vi "Create Spy.vi"(8 "error in (no error)":errorcluster) -> (0 "error out":errorcluster, 3 "LabSpy Out":refnum<data-value>)   [LabVIEW 2013, in "LabSpy.lvclass"]
doc: "Create a new spy object for use."
uses:
  LabSpy.lvclass
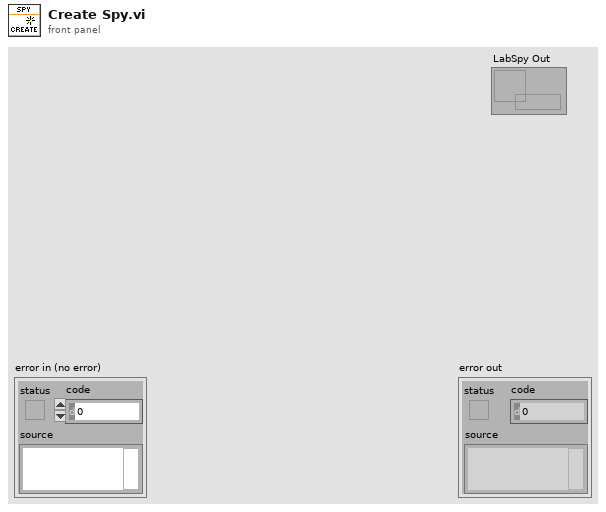
[diagram p1: front panel]
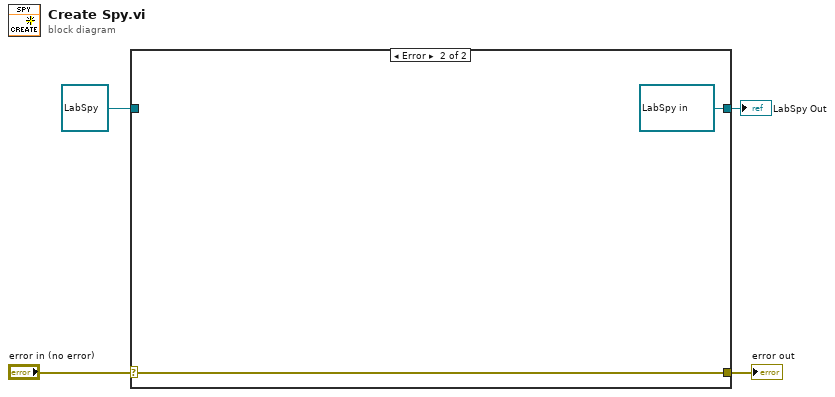
[diagram p0: block diagram]
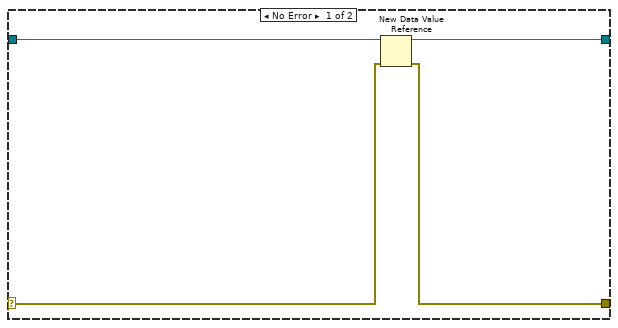
[diagram p2: hidden frame]
diagram:
  n1 = case shown="Error" "error in (no error)" {
    selector: "error in (no error)" -> [w5 w10]
    tunnel: [w6 w10] -> w3
    tunnel: [w7 refnum<data-value> refnum ("data value reference")] -> w1
    tunnel: refnum<class "LabSpy.lvclass"> refnum ("LabSpy in") -> [w8 _]
    frame No Error {
      n2 = New Data Value Reference(data value=w8, error in=w5) -> (data value reference=w7:refnum<data-value>, error out=w6:errorcluster)
    }
    frame Error {
    }
  }
  "error out" <- w3
  "LabSpy Out" <- w1
